vi "7XNN.vi"(11 "Variables and Memory in":T1 {"GFX" format="%02x"}) -> (3 "Variables and Memory out":T1 {"GFX" format="%02x"})   [LabVIEW 2021]
uses:
  Controls/ClusterF.ctl
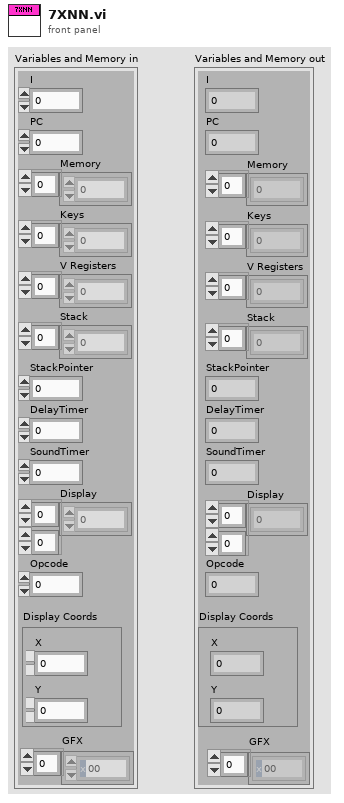
[diagram p1: front panel]
types:
  T1 = typedef "ClusterF.ctl" = cluster{"I":u16, "PC":u16, "Memory":u8[], "Keys":u8[], "V Registers":u8[], "Stack":u16[], "StackPointer":u16, "DelayTimer":u8, "SoundTimer":u8, "Display":u8[][], "Opcode":u16, "Display Coords":cluster{"X":u8, "Y":u8}, "GFX":u8[]}
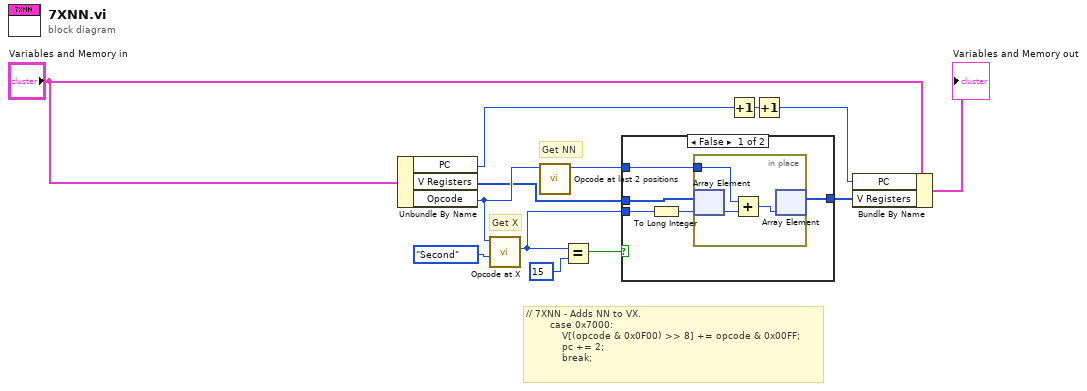
[diagram p0: block diagram]
diagram:
  # "// 7XNN - Adds NN to VX.\n        case 0x7000:\n            V[(opcode & 0x0F00) >> 8] += opcode & 0x00FF;\n            pc += 2;\n            break;"
  # "Get NN"
  # "Get X"
  n1 = Unbundle By Name("Variables and Memory in") -> ("PC"=w8:u16, "V Registers"=w3:u8[], "Opcode"=w13:u16)
  n2 = call "Opcode at X.vi"("X Position"=enum16{"First", "Second", "Third", "Fourth"}."Second", "Opcode"=w13) -> ("Opcode at X Position (U8)"=w11:u8)  [unwired: 9 in]
  n3 = call "Opcode at last 2 positions.vi"("Opcode"=w13) -> ("00FF"=w12:u8)  [unwired: 10 in]
  n4 = Equal?(x=w11, y=u8 15) -> (x = y?=w1:bool)
  n5 = case shown="False" w1 {
    tunnel: w3 -> [w18 w22]
    tunnel: w11 -> [w17 _]
    tunnel: w12 -> [w16 _]
    tunnel: [w15 w22] -> w6
    frame False {
      n6 = To Long Integer(number=w17) -> (32bit integer=w14:i32)
      n7 = in-place {
        in-place-border: w16 -> [w21]
        n8 = in-place-array #1(w18, w14) -> (w20:u8)
        n9 = Add(x=w21, y=w20) -> (x+y=w19:u8)
        n10 = in-place-array #1(w19) -> (w15:u8[])  [unwired: 1 out]
      }
    }
    frame True {
      # "Carry flag (VF) is not changed"
    }
  }
  n11 = Increment(x=w8) -> (x+1=w7:u16)
  n12 = Increment(x=w7) -> (x+1=w9:u16)
  n13 = Bundle By Name(cluster="Variables and Memory in", "PC"=w9, "V Registers"=w6) -> (→"Variables and Memory out":T1)
